vi "stop.vi"(8 "error in (no error)":errorcluster, 11 "HSDIO in":refnum<class "HSDIO.lvclass">) -> (0 "error out":errorcluster, 3 "HSDIO out":refnum<class "HSDIO.lvclass">)   [LabVIEW 2013, in "HSDIO.lvclass"]
uses:
  HSDIO.lvclass
  HSDIO.lvclass/HSDIO.ctl
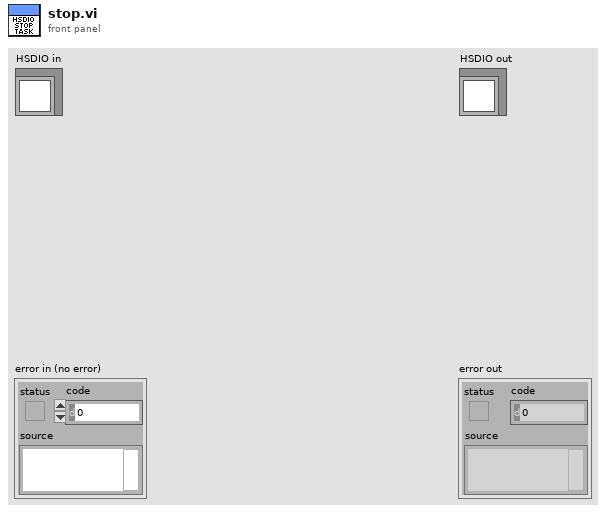
[diagram p1: front panel]
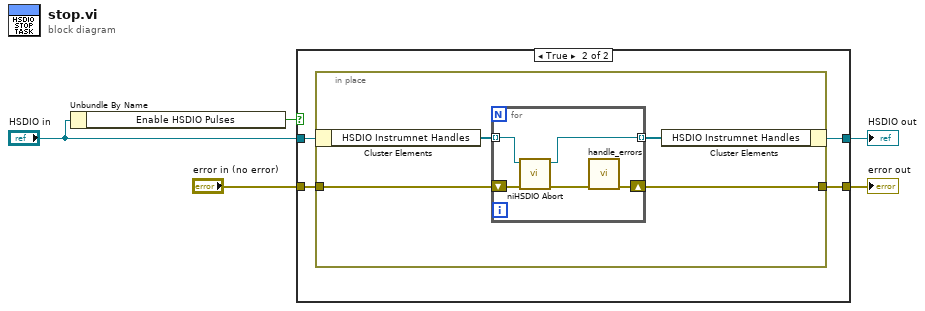
[diagram p0: block diagram]
diagram:
  n1 = Unbundle By Name("HSDIO in") -> ("Enable HSDIO Pulses"=w3:bool)
  n2 = case shown="True" w3 {
    tunnel: [w7 w8] -> w4
    tunnel: "error in (no error)" -> [w7 w11]
    tunnel: "HSDIO in" -> [w6 w10]
    tunnel: [w6 w9] -> w1
    frame False {
    }
    frame True {
      n3 = in-place {
        in-place-border: w11 -> [w15]
        in-place-border: [w14] -> w8
        n4 = in-place-cluster #1(w10) -> ("HSDIO Instrumnet Handles"=w13:refnum<k15>[])
        n5 = for {
          tunnel: w13 -> [w19] mode=indexing
          tunnel: [w18] -> w12 mode=indexing
          shift-right: [w16] -> w14
          shift-left: w15 -> [w20]
          n6 = call <instrlib>:"niHSDIO Abort.vi"("error in (no error)"=w20, "instrument handle"=w19) -> ("error out"=w17:errorcluster, "instrument handle out"=w18:refnum<k15>)  [unwired: 8 in]
          n7 = call "handle_errors.vi"("error in (no error)"=w17) -> ("error out"=w16:errorcluster)  [unwired: 14 in]
        }
        n8 = in-place-cluster #1("HSDIO Instrumnet Handles"=w12) -> (w9:refnum<class "HSDIO.lvclass">)
      }
    }
  }
  "error out" <- w4
  "HSDIO out" <- w1
